vi "Query Current Calibration.vi"(8 "error in (no error)":errorcluster, 11 "VNA-ENA in":refnum<class "VNA-ENA.lvclass">) -> (0 "error out":errorcluster, 3 "VNA-ENA out":refnum<class "VNA-ENA.lvclass">)   [LabVIEW 2020, in "VNA-ENA.lvclass"]
uses:
  VNA-ENA.lvclass
  C:/Sandbox/Git_Sandbox/WiSpry Test Framework source code (LV20)/WiSpry Test Framework/Instruments/Vector Network Analyzer/Vector Network Analyzer.lvclass
  C:/Sandbox/Git_Sandbox/WiSpry Test Framework source code (LV20)/WiSpry Test Framework/Instruments/Instrument.lvclass
  Instrument.lvclass/Instrument.ctl
  Vector Network Analyzer.lvclass/Vector Network Analyzer.ctl
  Instrument.lvclass
  Vector Network Analyzer.lvclass
panel:
  out "Calibration info":string
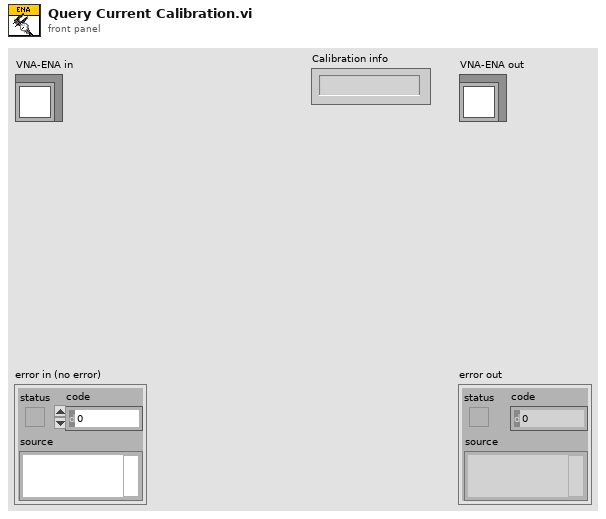
[diagram p1: front panel]
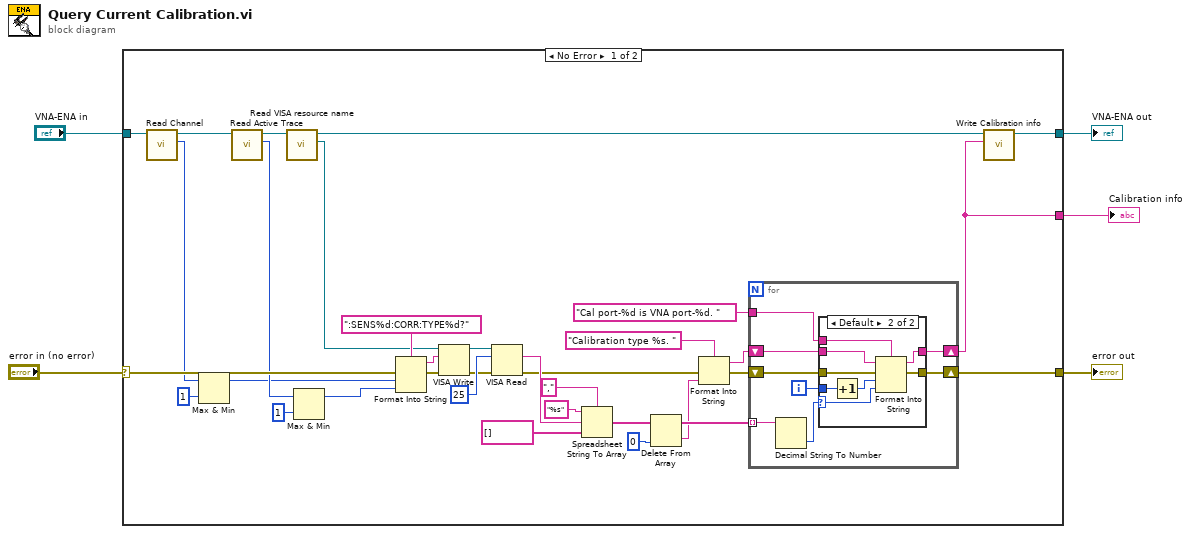
[diagram p0: block diagram]
diagram:
  n1 = case shown="No Error" "error in (no error)" {
    selector: "error in (no error)" -> [w20 w59]
    tunnel: [w19 w59] -> w4
    tunnel: "VNA-ENA in" -> [w15 w58]
    tunnel: [w18 w58] -> w2
    tunnel: [w6 _] -> w1
    frame No Error {
      n2 = call-dynamic "Read Channel.vi"("Vector Network Analyzer in"=w15) -> ("Channel"=w8:i32, "Vector Network Analyzer out"=w17:refnum<class "VNA-ENA.lvclass">)  [unwired: 9 in]
      n3 = Max & Min(x=w8, y=1) -> (max(x,y)=w7:i32)  [unwired: 1 out]
      n4 = call "Read Active Trace.vi"("Vector Network Analyzer in"=w17) -> ("Active Trace"=w10:u8, "Vector Network Analyzer out"=w13:refnum<class "VNA-ENA.lvclass">)  [unwired: 9 in]
      n5 = call "Read VISA resource name.vi"("Instrument in"=w13) -> ("VISA resource name"=w16:refnum<visa-resource-name>, "Instrument out"=w14:refnum<class "VNA-ENA.lvclass">)  [unwired: 9 in]
      n6 = Max & Min(x=w10, y=u8 1) -> (max(x,y)=w9:u8)  [unwired: 1 out]
      n7 = Format Into String(format string=":SENS%d:CORR:TYPE%d?", error in=w20, w7, w9) -> (resulting string=w24:string, error out=w27:errorcluster)  [unwired: 1 in]
      n8 = VISA Write(VISA resource name=w16, write buffer=w24, error in (no error)=w27) -> (VISA resource name out=w26:refnum<visa-resource-name>, error out=w25:errorcluster)  [unwired: 1 out]
      n9 = VISA Read(VISA resource name=w26, byte count=u32 25, error in (no error)=w25) -> (read buffer=w23:string, error out=w21:errorcluster)  [unwired: 2 out]
      n10 = Spreadsheet String To Array(delimiter (Tab)=",", format string="%s" ("delimiter (Tab)"), spreadsheet string=w23, array type (2D Dbl)=string[] []) -> (array=w34:string[])
      n11 = Delete From Array(array=w34, index=0) -> (deleted portion=w32:string, array with subset deleted=w33:string[])  [unwired: 1 in]
      n12 = Format Into String(format string="Calibration type %s. ", error in=w21, w32) -> (resulting string=w30:string, error out=w22:errorcluster)  [unwired: 1 in]
      n13 = for {
        tunnel: w33 -> [w46] mode=indexing
        tunnel: "Cal port-%d is VNA port-%d. " ("format string") -> [w47]
        shift-right: [w42] -> w6
        shift-left: w30 -> [w43]
        shift-right: [w40] -> w19
        shift-left: w22 -> [w41]
        i -> [w44]
        n14 = Decimal String To Number(string=w46) -> (number=w45:i32)  [unwired: 2 in, 1 out]
        n15 = case shown="Default" w45 {
          selector: w45 -> [_ w56]
          tunnel: w47 -> [_ w57]
          tunnel: w44 -> [_ w55]
          tunnel: w43 -> [w49 w53]
          tunnel: [w49 w52] -> w42
          tunnel: w41 -> [w48 w51]
          tunnel: [w48 w50] -> w40
          frame 0 {
          }
          frame Default {
            n16 = Increment(x=w55) -> (x+1=w54:i32)
            n17 = Format Into String(format string=w57, initial string=w53, error in=w51, w54, w56) -> (resulting string=w52:string, error out=w50:errorcluster)
          }
        }
      }
      n18 = call-dynamic "Write Calibration info.vi"("Calibration info"=w6, "Vector Network Analyzer in"=w14) -> ("Vector Network Analyzer out"=w18:refnum<class "VNA-ENA.lvclass">)  [unwired: 9 in]
    }
    frame Error {
    }
  }
  "error out" <- w4
  "VNA-ENA out" <- w2
  "Calibration info" <- w1
